vi "GetLibraryPath.vi"() -> (3 "GlobalDLLPath":path)   [LabVIEW 2020, in "AIM664LV.lvlib"]
uses:
  AIM664LV.lvlib
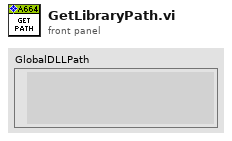
[diagram p1: front panel]
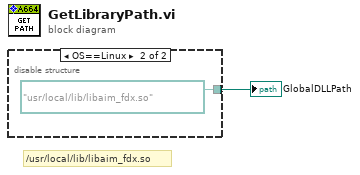
[diagram p0: block diagram]
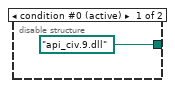
[diagram p2: hidden frame]
diagram:
  # "/usr/local/lib/libaim_fdx.so"
  n1 = disable-structure shown="OS==Linux" {
    disable-tunnel: [path "api_civ.9.dll" ("GlobalDLLPath") path "/usr/local/lib/libaim_fdx.so" ("DLL Path (if required)")] -> w1
    frame condition #0 (active) {
    }
    frame condition #1 {
    }
  }
  "GlobalDLLPath" <- w1
